vi "InitTables.vi"(8 "ErrorArray in":errorcluster[](array[cluster]), 10 "TableRefArray":refnum<vi>[](array[refnum]), 11 "IniFileRef in":T1) -> (0 "ErrorArray Out":errorcluster[](array[cluster]), 3 "IniFileRef out":T1)   [LabVIEW 2014, in "Ini_lib.lvlib"]
uses:
  Ini_lib.lvlib
  <vilib>/Utility/config.llb/Config Data RefNum.ctl
  typedefs/clTableData.ctl
  <userlib>/NIST/NISTErrorLib/NISTErrorLib.lvlib
  <vilib>/Utility/config.llb/NI_LVConfig.lvlib
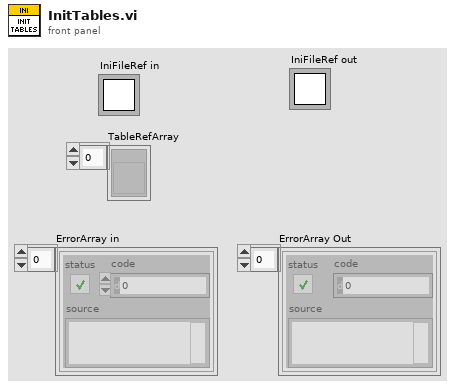
[diagram p1: front panel]
types:
  T1 = typedef "NI_LVConfig.lvlib/Config Data RefNum.ctl" = refnum<k1>
  T2 = typedef "Ini_lib.lvlib/clTableData.ctl" = cluster{"RowHdrs":string[], "ColHdrs":string[], "DefaultParams":string[][]}
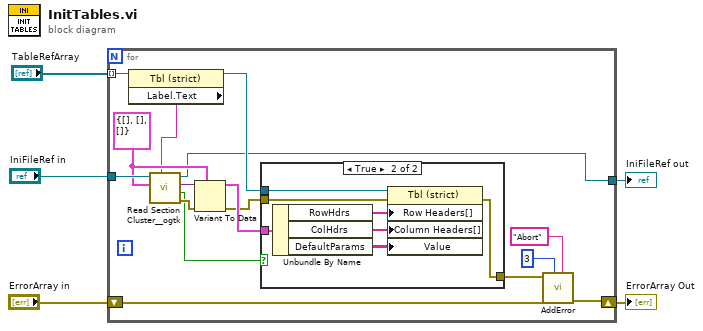
[diagram p0: block diagram]
diagram:
  n1 = for {
    tunnel: "TableRefArray" -> [w16] mode=indexing
    tunnel: "IniFileRef in" -> [w19]
    tunnel: [w12] -> w1
    shift-right: [w10] -> w5
    shift-left: "ErrorArray in" -> [w11]
    w18 = T2 {"RowHdrs"=[], "ColHdrs"=[], "DefaultParams"=[]} ("ParamsHdrs")
    n2 = property class="Tbl (strict)"(reference=w16) -> (reference out=w14:refnum<vi>, "Label.Text"=w15:string)  [unwired: 1 in, 1 out]
    n3 = call <userlib>:"Read Section Cluster__ogtk.vi"("section (optional)"=w15, "Section Formatted Cluster Type"=w18, "refnum"=w19) -> ("error out"=w21:errorcluster, "all found?"=w6:bool, "Section Formatted Cluster"=w20:variant, "dup refnum"=w12:T1)  [unwired: 4 in, 1 out]
    n4 = Variant To Data(error in=w21, type=w18, Variant=w20) -> (data=w17:T2, error out=w13:errorcluster)
    n5 = case shown="True" w6 {
      tunnel: w17 -> [_ w29]
      tunnel: w14 -> [_ w27]
      tunnel: w13 -> [w22 w26]
      tunnel: [w22 w25] -> w9
      frame False {
      }
      frame True {
        n6 = Unbundle By Name(w29) -> ("RowHdrs"=w23:string[], "ColHdrs"=w24:string[], "DefaultParams"=w28:string[][])
        n7 = property on="Property Node" class="Tbl (strict)"(reference=w27, error in=w26, "Row Headers[]"=w23, "Column Headers[]"=w24, "Value"=w28) -> (error out=w25:errorcluster)  [unwired: 1 out]
      }
    }
    n8 = call <userlib>:"AddError.vi"("Severity"="Abort", "Priority"=u8 3, "ErrorArray"=w11, "error in (no error)"=w9) -> ("ErrorArray"=w10:errorcluster[])  [unwired: 6 in, 1 out]
  }
  "ErrorArray Out" <- w5
  "IniFileRef out" <- w1
